vi "Set Auth URL.vi"(10 "Auth URL":string, 11 "OAuth2 in":refnum<class "OAuth2.lvclass">) -> (3 "OAuth2 out":refnum<class "OAuth2.lvclass">)   [LabVIEW 2020, in "OAuth2.lvlib" / "OAuth2.lvclass"]
uses:
  OAuth2.lvclass
  OAuth2.lvclass/OAuth2.ctl
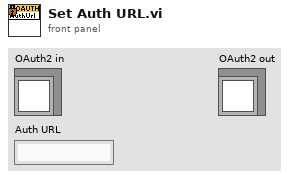
[diagram p1: front panel]
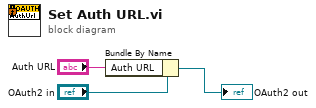
[diagram p0: block diagram]
diagram:
  n1 = Bundle By Name(cluster="OAuth2 in", "Auth URL"="Auth URL") -> (→"OAuth2 out":refnum<class "OAuth2.lvclass">)
